vi "Remote Mode--SubVI.vi"(4 "Instance":i32=1, 8 "error in":errorcluster, 9 "Mode (Auto)":u16(ring)=10 items=["Auto"=10, "Manual"=54], 10 "Enable (T)":bool=TRUE, 11 "Watlow F4T in":refnum<class "Watlow F4T.lvclass">) -> (0 "error out":errorcluster, 3 "Watlow F4T out":refnum<class "Watlow F4T.lvclass">)   [LabVIEW 2024, in "Watlow F4T.lvclass"]
uses:
  Watlow F4T.lvclass
  Private/Controls/Standard Bus Commands--Enum.ctl
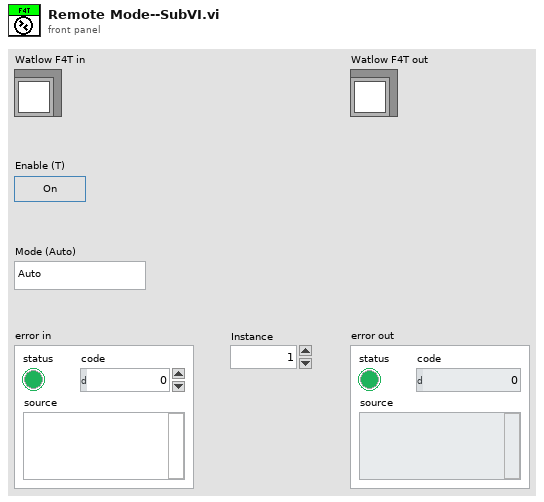
[diagram p1: front panel]
types:
  T1 = typedef "Watlow F4T.lvclass/Standard Bus Commands--Enum.ctl" = enum16{"Remote Setpoint", "Remote Mode", "Temp Feedback", "Target Setpoint", "Current Setpoint", "Setpoint Lower Limit", "Setpoint Upper Limit", "Ramp Rate Y", "Ramp Rate X", "Ramp Rate Action", "Temp Control State", "Temp Control Mode", "Power", "Heat Power", "Cool Power"}
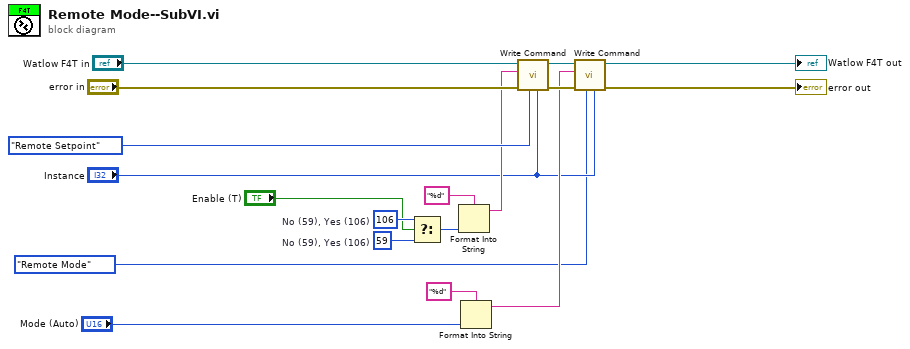
[diagram p0: block diagram]
diagram:
  w13 = 59  # No (59), Yes (106)
  w14 = 106  # No (59), Yes (106)
  n1 = Select(t=w14, s="Enable (T)", f=w13) -> (s? t:f=w12:i32)
  n2 = Format Into String(format string="%d", w12) -> (resulting string=w11:string)  [unwired: 2 in, 1 out]
  n3 = Format Into String(format string="%d", "Mode (Auto)") -> (resulting string=w4:string)  [unwired: 2 in, 1 out]
  n4 = call "Write Command.vi"("Instance"="Instance", "Commands"=Standard_Bus_Commands--Enum."Remote Setpoint", "error in (no error)"="error in", "Set Value"=w11, "Watlow F4T In"="Watlow F4T in") -> ("error out"=w5:errorcluster, "Watlow F4T out"=w8:refnum<class "Watlow F4T.lvclass">)  [unwired: 5 in]
  n5 = call "Write Command.vi"("Instance"="Instance", "Commands"=Standard_Bus_Commands--Enum."Remote Mode", "error in (no error)"=w5, "Set Value"=w4, "Watlow F4T In"=w8) -> ("error out"=→"error out":errorcluster, "Watlow F4T out"=→"Watlow F4T out":refnum<class "Watlow F4T.lvclass">)  [unwired: 5 in]
